vi "U3 Stream with FFT.vi"() -> ()   [LabVIEW 2021]
uses:
  <vilib>/Analysis/NI_AALPro.lvlib
panel:
  out "RMS Voltage vs. Frequency":cluster{i32, dbl, dbl[][]}(graph)
  in  "Scan List (-)":u8[](array[numeric])=[31, 31, 31, 31, 31, 31, 31, 31, 31, 31, 31, 31, 31, 31, 31, 31, 31, 31, 31, 31, 31, 31, 31, 31, 31, 31, 31, 31, 31, 31, 31, 31, 31, 31, 31, 31, 31, 31, 31, 31, 31, 31, 31, 31, 31, 31, 31, 31, 31, 31, 31, 31, 31, 31, 31, 31, 31, 31, 31, 31, 31, 31, 31, 31, 31, 31, 31, 31, 31, 31, 31, 31, 31, 31, 31, 31, 31, 31, 31, 31, 31, 31, 31, 31, 31, 31, 31, 31, 31, 31, 31, 31, 31, 31, 31, 31, 31, 31, 31, 31, 31, 31, 31, 31, 31, 31, 31, 31, 31, 31, 31, 31, 31, 31, 31, 31, 31, 31, 31, 31, 31, 31, 31, 31, 31, 31, 31, 31]
  out "Voltage vs. Time":cluster{i32, dbl, dbl[][]}(graph)
  in  "Scan List (+)":u8[](array[numeric])=[0, 1]
  out "Actual Scan Rate (Hz)":dbl format="%.3f"
  out "# Scans Read":i32
  out "# of iterations":i32
  out "Data":dbl[][](array[numeric]) format="%.3f"
  in  "Scan Rate (Hz)":dbl=1024.0 format="%.3f"
  in  "stop":bool
  out "Error Message":string
  # "This example streams from the first found USB U3.  Streaming\nrequires U3 hardware revision 1.21+."
  # "The + scan list is the positive\nchannels.  For each element in\nthe + list, there must also be\nan element in the - list, which is\nthe negative channels.  For\nsingle-ended channels, put in\n31 for the negative channel."
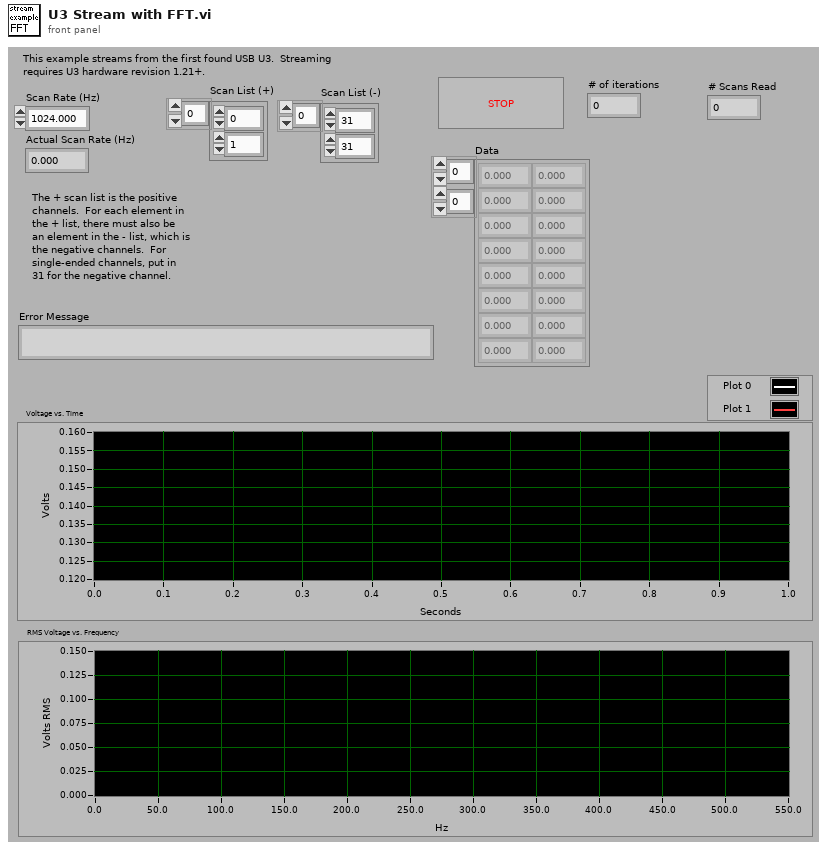
[diagram p1: front panel]
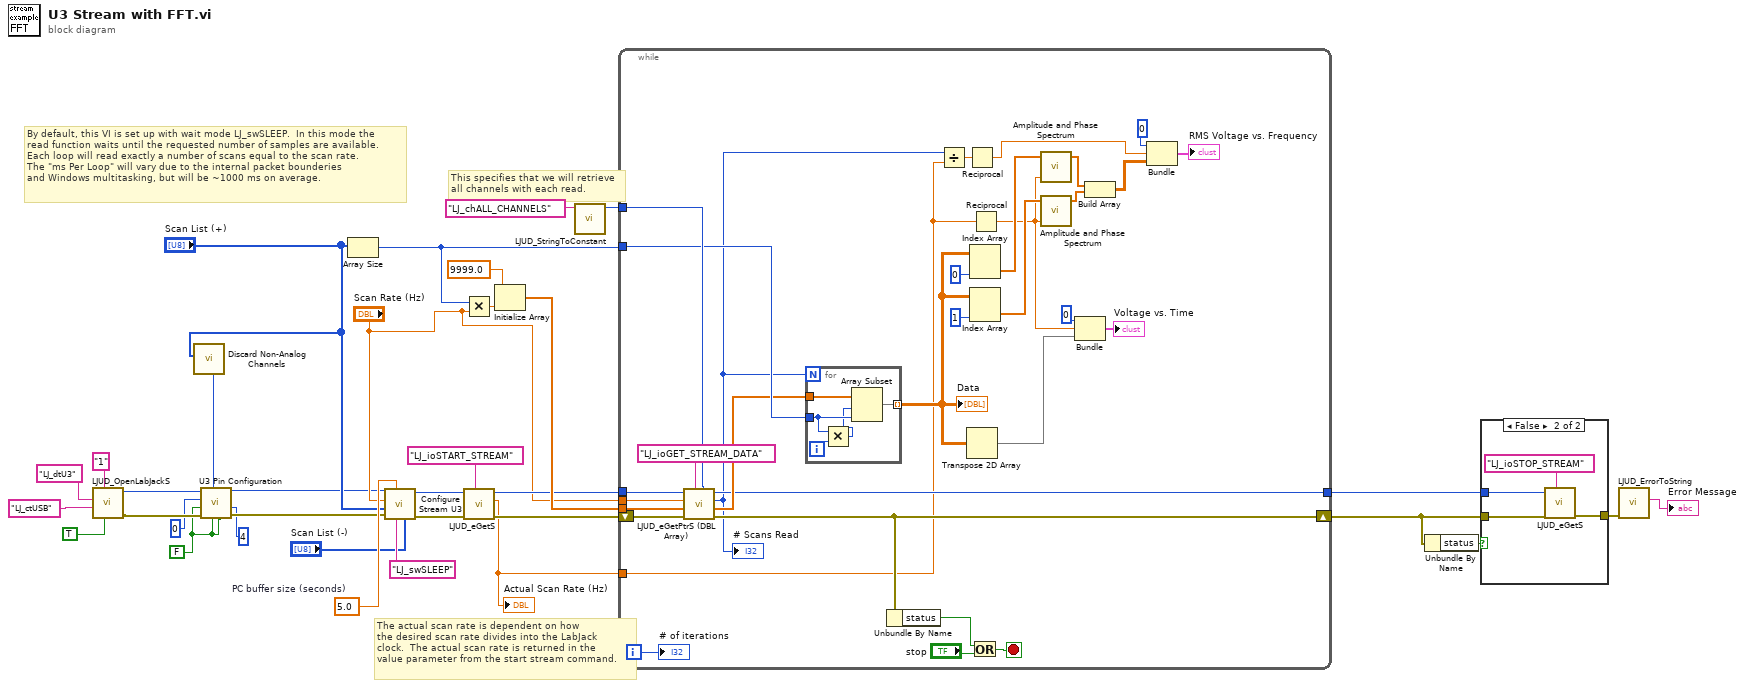
[diagram p0: block diagram]
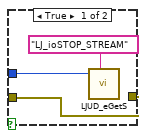
[diagram p2: hidden frame]
diagram:
  w12 = FALSE ("Enable DAC1")
  w24 = 5.0  # PC buffer size (seconds)
  # "This specifies that we will retrieve\nall channels with each read."
  # "The actual scan rate is dependent on how\nthe desired scan rate divides into the LabJack\nclock.  The actual scan rate is returned in the\nvalue parameter from the start stream command."
  # "By default, this VI is set up with wait mode LJ_swSLEEP.  In this mode the\nread function waits until the requested number of samples are available.\nEach loop will read exactly a number of scans equal to the scan rate.\nThe \"ms Per Loop\" will vary due to the internal packet bounderies\nand Windows multitasking, but will be ~1000 ms on average."
  n1 = call "LJUD_OpenLabJackS.vi"("FirstFound"=TRUE, "Address"="1", "ConnectionType"="LJ_ctUSB", "DeviceType"="LJ_dtU3") -> ("error out"=w15:errorcluster, "Handle"=w16:i32)  [unwired: 5 in, 1 out]
  n2 = call "Discard Non-Analog Channels.vi"("Channels In"="Scan List (+)") -> ("FIO/EIO Analog Enable"=w11:i32)  [unwired: 7 in, 3 out]
  n3 = call "U3 Pin Configuration.vi"("Timer/Counter Pin Offset"=u8 4, "Enable Counter1"=w12, "Enable Counter0"=w12, "FIO/EIO Analog Enable"=w11, "error in"=w15, "Enable DAC1"=w12, "Number of Timers Enabled"=u8 0, "Handle In"=w16) -> ("error out"=w8:errorcluster, "Handle Out"=w9:i32)  [unwired: 2 in]
  n4 = Array Size(array="Scan List (+)") -> (size(s)=w28:i32)
  n5 = call "Configure Stream U3.vi"("Scan List (-)"="Scan List (-)", "Wait Mode"="LJ_swSLEEP" ("Wait Mode (2)"), "PC buffer size (seconds)"=w24, "error in"=w8, "Scan List (+)"="Scan List (+)", "Scan Rate (Hz)"="Scan Rate (Hz)", "Handle In"=w9) -> ("error out"=w32:errorcluster, "Handle Out"=w33:i32)  [unwired: 2 in, 1 out]
  n6 = Multiply(x=w28, y="Scan Rate (Hz)") -> (x*y=w31:dbl)
  n7 = call "LJUD_eGetS.vi"("IOType"="LJ_ioSTART_STREAM", "error in"=w32, "Handle In"=w33) -> ("error out"=w18:errorcluster, "Value Read"=w1:dbl, "Handle Out"=w23:i32)  [unwired: 6 in]
  "Actual Scan Rate (Hz)" <- w1
  n8 = Initialize Array(9999.0, w31) -> (w29:dbl[])
  n9 = call "LJUD_StringToConstant.vi"("String"="LJ_chALL_CHANNELS") -> ("Constant Number"=w19:i32)  [unwired: 9 in, 1 out]
  n10 = while {
    tunnel: w1 -> [w40]
    tunnel: [w53] -> w5
    shift-left: w18 -> [w57]
    shift-right: [w54] -> w17
    tunnel: w19 -> [w58]
    tunnel: w28 -> [w56]
    tunnel: w29 -> [w61]
    tunnel: "Scan Rate (Hz)" -> [w60]
    tunnel: w23 -> [w63]
    i -> [w59]
    stop <- w64 stop-if-true
    n11 = call "LJUD_eGetPtrS (DBL Array).vi"("Channel"=w58, "IOType"="LJ_ioGET_STREAM_DATA", "error in"=w57, "DBL Array Write"=w61, "Value"=w60, "Handle In"=w63) -> ("error out"=w54:errorcluster, "DBL Array Read"=w55:dbl[], "Value"=w39:i32, "Handle Out"=w53:i32)  [unwired: 2 in]
    "# Scans Read" <- w39
    n12 = for {
      N: w39 -> [_]
      tunnel: w55 -> [w71]
      tunnel: w56 -> [w70]
      tunnel: [w67] -> w41 mode=indexing
      i -> [w69]
      n13 = Multiply(x=w70, y=w69) -> (x*y=w68:i32)
      n14 = Array Subset(array=w71, index=w68, length=w70) -> (w67:dbl[])
    }
    "Data" <- w41
    n15 = Unbundle By Name(w54) -> ("status"=w65:bool)
    n16 = Divide(x=w39, y=w40) -> (x/y=w49:dbl)
    n17 = Reciprocal(x=w49) -> (1/x=w46:dbl)
    n18 = Transpose 2D Array(2D array=w41) -> (transposed array=w36:dbl[][])
    n19 = Index Array(array=w41, index (col)=0 ("Index")) -> (element=w45:dbl[])  [unwired: 1 in]
    n20 = Index Array(array=w41, index (col)=1 ("Index")) -> (element=w50:dbl[])  [unwired: 1 in]
    n21 = Or(x=w65, y="stop") -> (x .or. y?=w64:bool)
    n22 = Reciprocal(x=w40) -> (1/x=w37:dbl)
    n23 = call <vilib>:"Amplitude and Phase Spectrum.vi"("dt"=w37, "Signal (V)"=w45) -> ("Amp Spectrum Mag (Vrms)"=w44:dbl[])  [unwired: 1 in, 2 out]
    n24 = call <vilib>:"Amplitude and Phase Spectrum.vi"("dt"=w37, "Signal (V)"=w50) -> ("Amp Spectrum Mag (Vrms)"=w48:dbl[])  [unwired: 1 in, 2 out]
    n25 = Bundle(0, w37, w36) -> (→"Voltage vs. Time":cluster{i32, dbl, dbl[][]})  [unwired: 1 in]
    n26 = Build Array(w44, w48) -> (w43:dbl[][])
    n27 = Bundle(0, w46, w43) -> (→"RMS Voltage vs. Frequency":cluster{i32, dbl, dbl[][]})  [unwired: 1 in]
    "# of iterations" <- w59
  }
  n28 = Unbundle By Name(w17) -> ("status"=w21:bool)
  n29 = case shown="False" w21 {
    tunnel: [w73 w77] -> w26
    tunnel: w17 -> [w73 w76]
    tunnel: w5 -> [w72 w75]
    frame True {
      n30 = call "LJUD_eGetS.vi"("IOType"="LJ_ioSTOP_STREAM", "Handle In"=w72) -> ()  [unwired: 7 in, 3 out]
    }
    frame False {
      n31 = call "LJUD_eGetS.vi"("IOType"="LJ_ioSTOP_STREAM", "error in"=w76, "Handle In"=w75) -> ("error out"=w77:errorcluster)  [unwired: 6 in, 2 out]
    }
  }
  n32 = call "LJUD_ErrorToString.vi"("error in"=w26) -> ("String"=→"Error Message":string)  [unwired: 10 in]
